vi "BRig_dataLC_Cue2_PostR_DelayOpt_l1.vi"() -> (2 "output_Cue2_PostR_DelayOpt":i32)   [LabVIEW 2014]
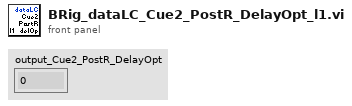
[diagram p1: front panel]
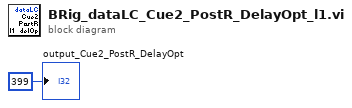
[diagram p0: block diagram]
diagram:
  "output_Cue2_PostR_DelayOpt" <- 399 ("output_iBlock")
